vi "Remove_unnecessary_groups.vi"() -> ()   [LabVIEW 2013]
uses:
  <vilib>/addons/h5labview/H5F_mode.ctl
  <userlib>/_OpenG.lib/file/file.llb/File Exists - Scalar__ogtk.vi
  <vilib>/addons/database/_DB Variant To Data/Database Variant To Data.xnode
  <vilib>/addons/h5labview/H5File.lvlib
  <vilib>/addons/h5labview/H5Base.lvlib
panel:
  out "Slide":dbl(slide) scale=0.0..100.0
  out "error out":errorcluster
  in  "error in (no error)":errorcluster
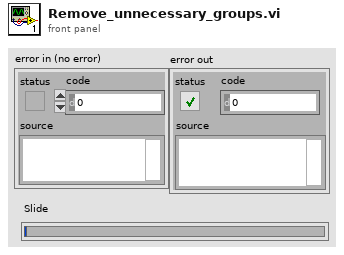
[diagram p1: front panel]
types:
  T1 = typedef "H5File.lvlib/H5F_mode.ctl" = enum16{"read-only", "read-write", "overwrite", "create new", "open or create"}
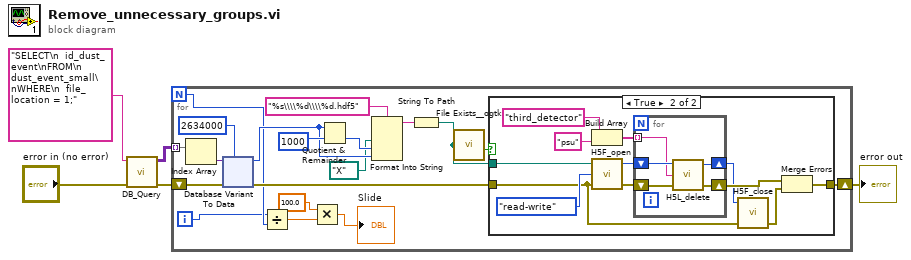
[diagram p0: block diagram]
diagram:
  n1 = call "DB_Query.vi"("error in (no error)"="error in (no error)", "Parameterized Query"="SELECT\n  id_dust_event\nFROM\n  dust_event_small\nWHERE\n  file_location = 1;") -> ("error out"=w4:errorcluster, "Results"=w2:variant[][])  [unwired: 7 in, 1 out]
  n2 = for {
    N -> [w10]
    shift-right: [w20] -> w5
    shift-left: w4 -> [w18]
    tunnel: w2 -> [w13] mode=indexing
    i -> [w9]
    n3 = Index Array(array=w13) -> (element=w19:variant)  [unwired: 1 in]
    n4 = xnode "Database Variant To Data"("database variant"=w19, "error in (no error)"=w18, "type"=i64 2634000) -> ("data"=w12:i64, "error out"=w14:errorcluster)
    n5 = Divide(x=w9, y=w10) -> (x/y=w8:dbl)
    n6 = Multiply(x=100.0, y=w8) -> (x*y=→"Slide":dbl)
    n7 = Quotient & Remainder(x=w12, y=1000) -> (floor(x/y)=w24:i64)  [unwired: 1 out]
    n8 = Format Into String(format string="%s\\\\%d\\\\%d.hdf5", path "X:/" ("Waveforms Path"), w24, w12) -> (resulting string=w17:string)  [unwired: 2 in, 1 out]
    n9 = String To Path(string=w17) -> (path=w16:path)
    n10 = call-poly <userlib>:"File Exists__ogtk.vi"("file path"=w16) -> ("exists"=w21:bool)  [unwired: 6 in, 1 out]
    n11 = case shown="True" w21 {
      tunnel: w16 -> [_ w67]
      tunnel: w14 -> [w57 w66]
      tunnel: [w57 w58] -> w20
      frame False {
      }
      frame True {
        n12 = Build Array("third_detector" ("name"), "psu" ("name")) -> (w59:string[])
        n13 = call <vilib>:"H5F_open.vi"("error in (no error)"=w66, "mode"=H5F_mode."read-write", "path"=w67) -> ("error out"=w65:errorcluster, "ref"=w61:i32)  [unwired: 1 in]
        n14 = for {
          shift-right: [w70] -> w64
          shift-left: w65 -> [w73]
          shift-right: [w71] -> w63
          shift-left: w61 -> [w74]
          tunnel: w59 -> [w72] mode=indexing
          n15 = call <vilib>:"H5L_delete.vi"("error in (no error)"=w73, "obj_name"=w72, "loc_id"=w74) -> ("error out"=w70:errorcluster, "loc_id out"=w71:i32)  [unwired: 1 in]
        }
        n16 = call <vilib>:"H5F_close.vi"("error in (no error)"=w66, "ref"=w63) -> ("error out"=w68:errorcluster)  [unwired: 3 in]
        n17 = Merge Errors(w64, w68) -> (w58:errorcluster)
      }
    }
  }
  "error out" <- w5
